vi "ECAT Download Error Handle.vi"(8 "error in":errorcluster) -> (0 "error out":errorcluster)   [LabVIEW 2019, in "SEECD System Explorer.lvlib"]
uses:
  <vilib>/Utility/error.llb/DialogType.ctl
  SEECD System Explorer.lvlib
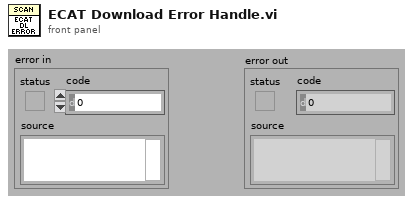
[diagram p1: front panel]
types:
  T1 = typedef "DialogType.ctl" = u16
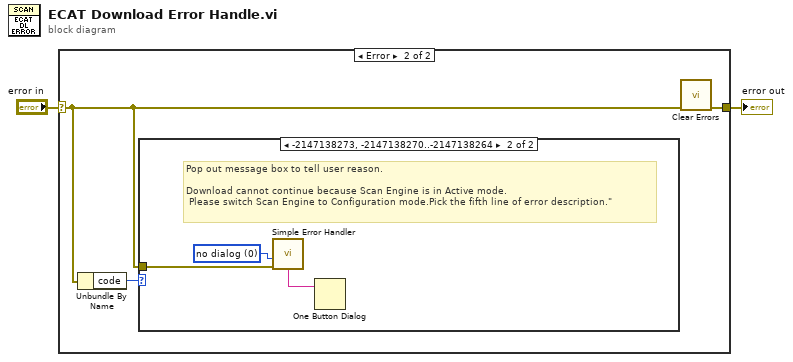
[diagram p0: block diagram]
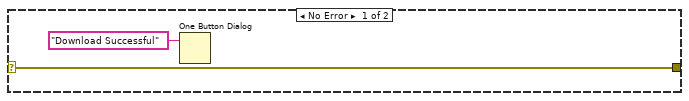
[diagram p2: hidden frame]
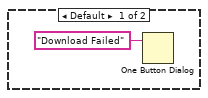
[diagram p3: hidden frame]
diagram:
  n1 = case shown="Error" "error in" {
    selector: "error in" -> [w3 w5]
    tunnel: [w3 w7] -> w2
    frame No Error {
      n2 = One Button Dialog(message="Download Successful") -> ()  [unwired: 2 out]
    }
    frame Error {
      n3 = Unbundle By Name(w5) -> ("code"=w6:i32)
      n4 = case shown="-2147138273, -2147138270..-2147138264" w6 {
        tunnel: w5 -> [_ w11]
        frame Default {
          n5 = One Button Dialog(message="Download Failed") -> ()  [unwired: 2 out]
        }
        frame -2147138273, -2147138270..-2147138264 {
          w10 = T1 0 items=["no dialog", "OK message", "continue or stop message", "OK message + warnings", "continue/stop + warnings"] ("type of dialog (OK msg:1)")
          # "Pop out message box to tell user reason.\n\nDownload cannot continue because Scan Engine is in Active mode.\n Please switch Scan Engine to Configuration mode.Pick the fifth line of error description.\""
          n6 = call <vilib>:"Simple Error Handler.vi"("type of dialog (OK msg:1)"=w10, "error in (no error)"=w11) -> ("message"=w9:string)  [unwired: 3 in, 4 out]
          n7 = One Button Dialog(message=w9) -> ()  [unwired: 1 in, 1 out]
        }
      }
      n8 = call <vilib>:"Clear Errors.vi"("error in (no error)"=w5) -> ("error out"=w7:errorcluster)  [unwired: 1 in, 5 out]
    }
  }
  "error out" <- w2
